vi "Output_file_Panel.vi"(8 "Show panel ?":bool, 9 "Channel Names":string[](array[string]), 10 "Header":string, 11 "Output filename":path=path "/G3_3 HD/Users/Paul/New Disp DB file") -> (0 "Save Full Res Data?":bool, 1 "Desired Columns":i32[](array[numeric]), 2 "Header Out":string, 3 "Output filename Out":path=path "/G3_3 HD/Users/Paul/New Disp DB file", 4 "Channels to Tabulate in header Out":i32[](listbox), 5 "Save Plotted rows only?":bool, 6 "Summarise mode":T1(ring), 7 "Grouping info":T3[](array[typedef]))   [LabVIEW 2010]
uses:
  Controls/Group_Binning.ctl
  Results_plotter_Global.vi
panel:
  in  "Channels to Tabulate in header":i32[](listbox)
  in  "Channels to first \"bin\" then output":i32[](listbox)
  in  "Channels to Ouput":i32[](listbox)
  out "Specified by Template":bool[](array[boolean])
  in  "Channel to bin":T2(array[cluster])
  in  "Summarize data":i32(listbox)=2
  in  "OK Button":bool
  in  "Column Selector":i32(listbox)
  in  "Row Selector":i32(listbox)=1
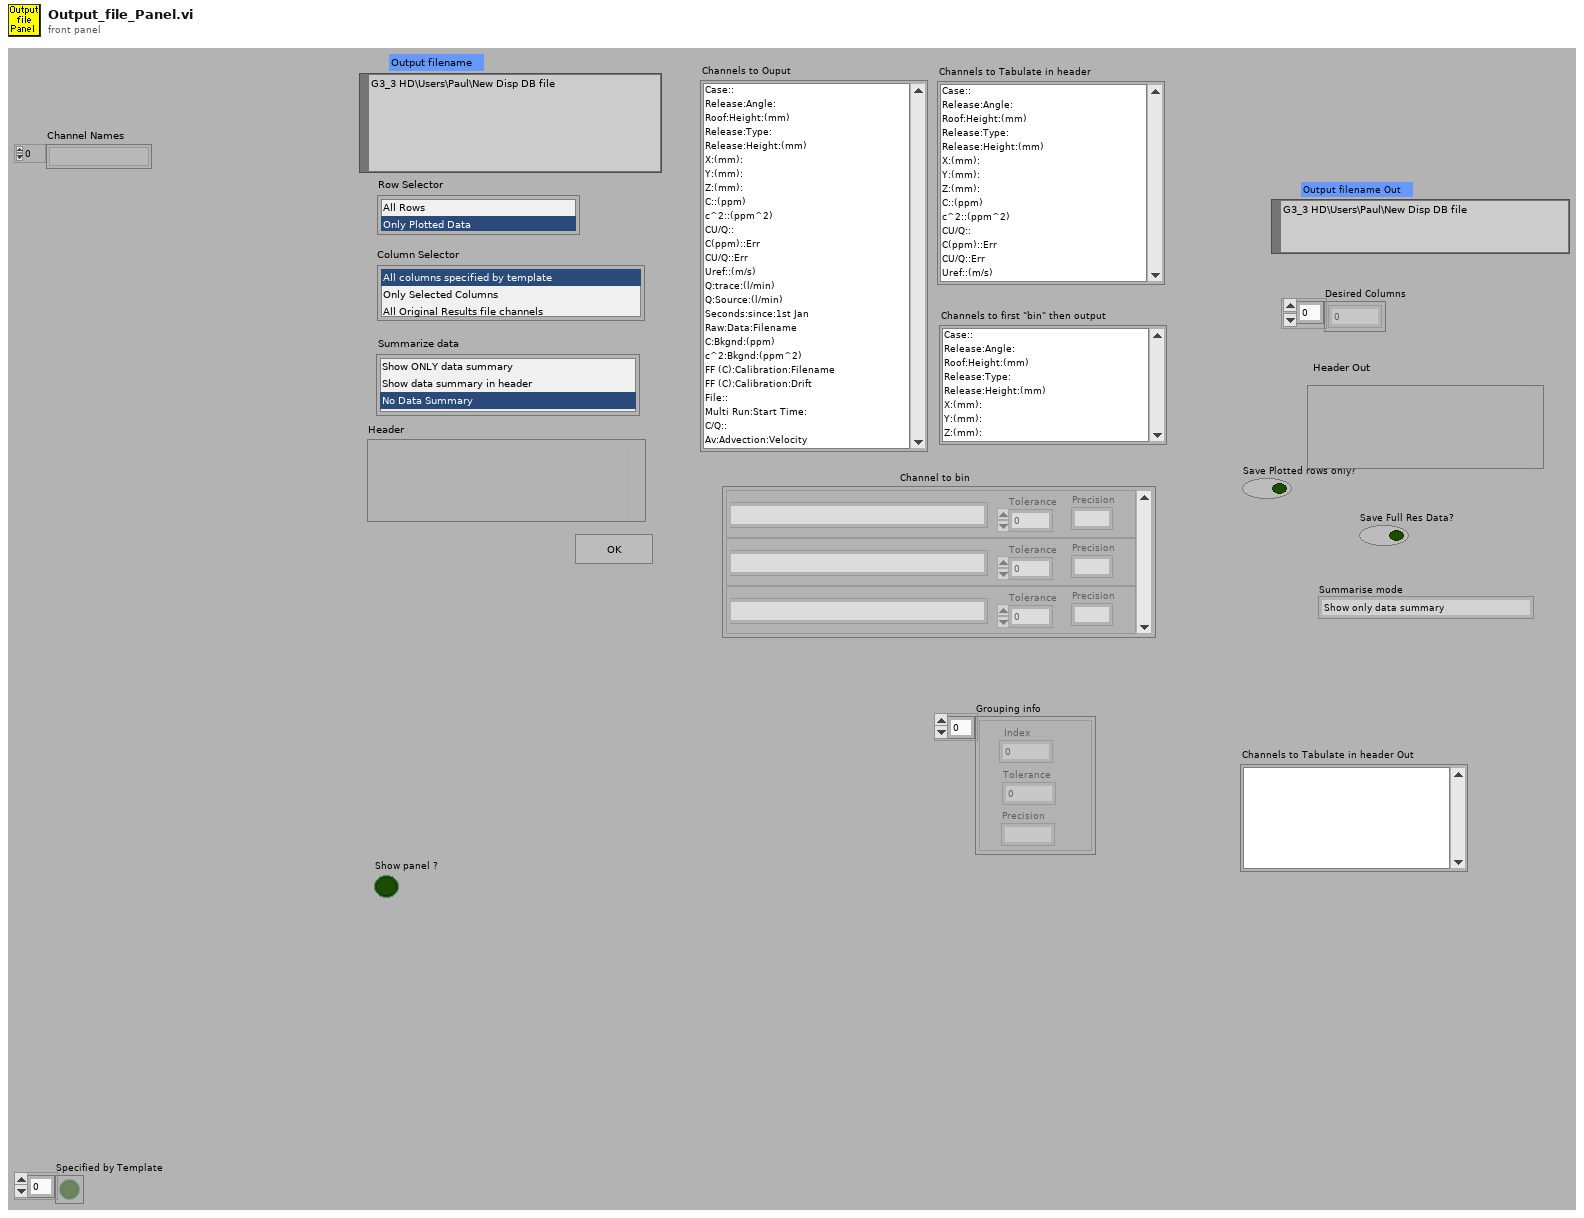
[diagram p1: front panel]
types:
  T1 = enum16{"Show only data summary", "Show data summary", "No data summary"}
  T2 = cluster{"Ch Name":string, "Tolerance":dbl, "Precision":string}[]
  T3 = typedef "Group_Binning.ctl" = cluster{"Index":i32, "Tolerance":dbl, "Precision":string}
  T4 = cluster{"Ch Name":string, "Tolerance":dbl, "Precision":string}
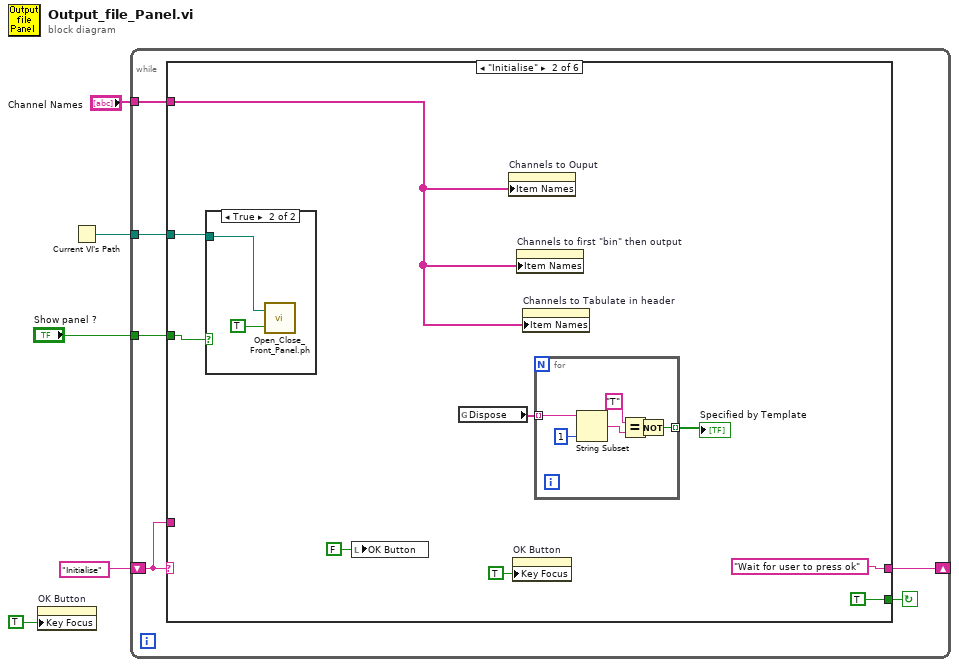
[diagram p0: block diagram]
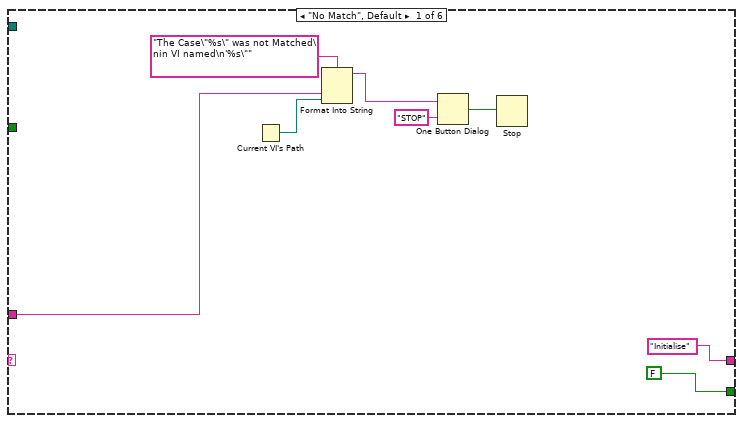
[diagram p2: hidden frame]
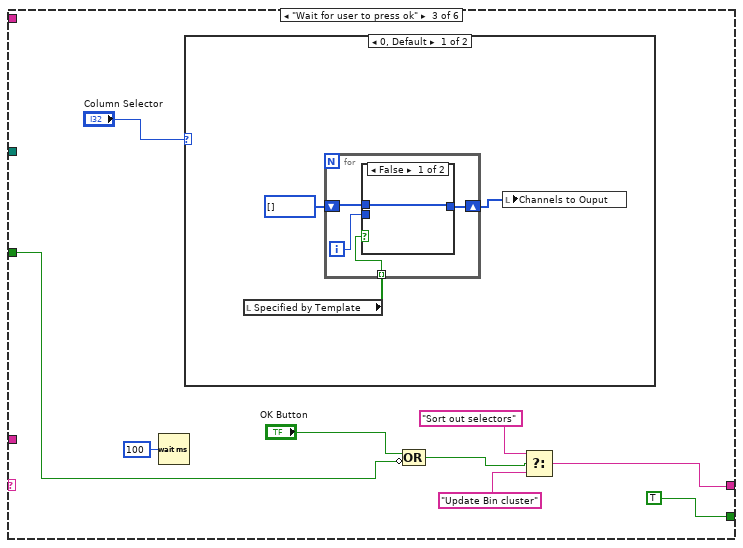
[diagram p4: hidden frame]
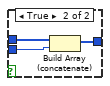
[diagram p5: hidden frame]
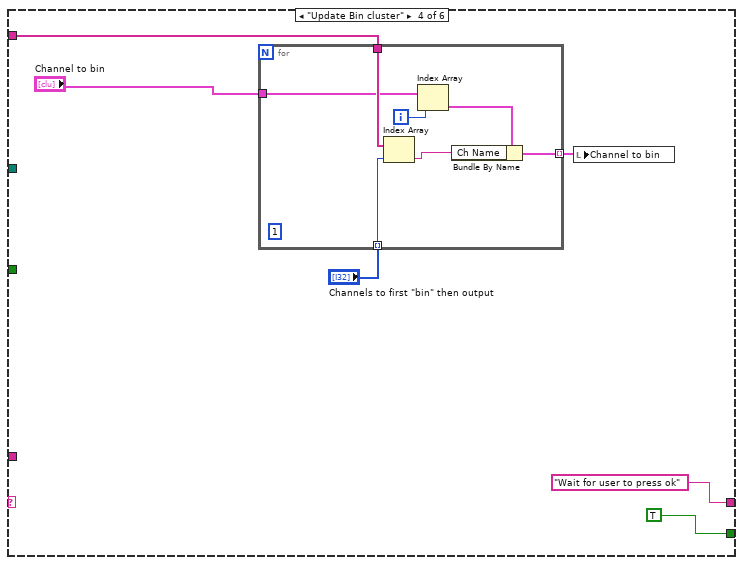
[diagram p7: hidden frame]
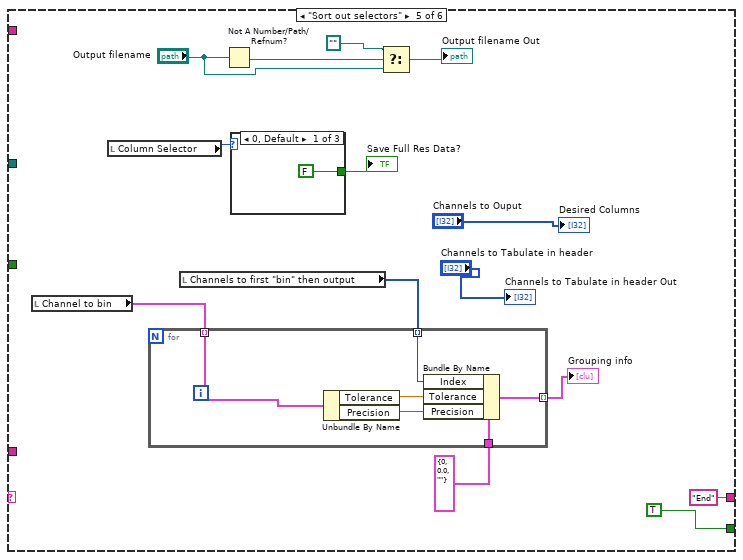
[diagram p8: hidden frame]
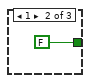
[diagram p9: hidden frame]
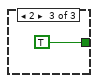
[diagram p10: hidden frame]
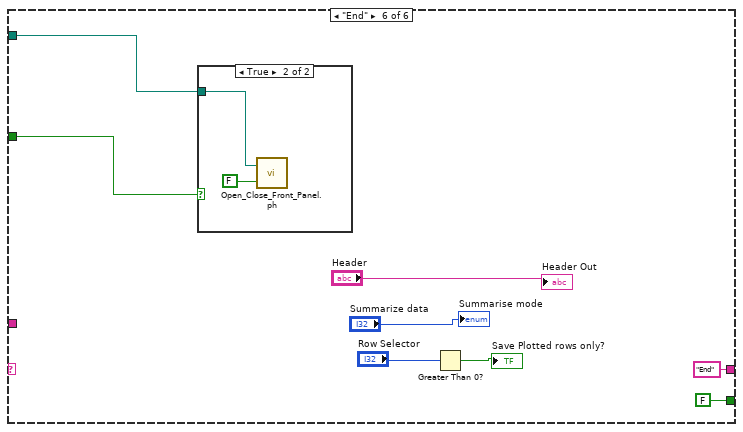
[diagram p11: hidden frame]
diagram:
  n1 = property on="OK Button" class="Bool (strict)"("Key Focus"=TRUE) -> ()  [unwired: 2 in, 2 out]
  n2 = Current VI's Path() -> (path=w3:path)
  n3 = while {
    shift-left: "Initialise" -> [w9]
    shift-right: [w10] -> _
    tunnel: "Show panel ?" -> [w8]
    tunnel: w3 -> [w7]
    tunnel: "Channel Names" -> [w6]
    stop <- w11 continue-if-true
    n4 = case shown="\"Initialise\"" w9 {
      tunnel: [FALSE TRUE TRUE TRUE TRUE FALSE] -> w11
      tunnel: ["Initialise" "Wait for user to press ok" w43 "Wait for user to press ok" "End" ("t") "End"] -> w10
      tunnel: w9 -> [w14 _ _ _ _ _]
      tunnel: w8 -> [_ w22 w37 _ _ w98]
      tunnel: w7 -> [_ w23 _ _ _ w97]
      tunnel: w6 -> [_ w24 _ w59 _ _]
      frame "No Match", Default {
        n5 = Current VI's Path() -> (path=w13:path)
        n6 = Format Into String(format string="The Case\"%s\" was not Matched\nin VI named\n'%s\"" ("Format String"), w14, w13) -> (resulting string=w17:string)  [unwired: 2 in, 1 out]
        n7 = One Button Dialog(message=w17, button name ("OK")="STOP") -> (true=w15:bool)
        n8 = Stop(stop? (T)=w15) -> ()
      }
      frame "Initialise" {
        n9 = case shown="True" w22 {
          tunnel: w23 -> [_ w30]
          frame False {
          }
          frame True {
            n10 = call "Open_Close_Front_Panel.ph.vi"("Front Panel Window:Open"=TRUE, "VI path"=w30) -> ()  [unwired: 2 out]
          }
        }
        n11 = local write "OK Button"(FALSE ("OK Button")) -> ()
        n12 = global read "Results_plotter_Global.vi" "Dispose"() -> (w28:string[])
        n13 = property on="Channels to Ouput" class="LstBox (strict)"("Item Names"=w24) -> ()  [unwired: 2 in, 2 out]
        n14 = property on="OK Button" class="Bool (strict)"("Key Focus"=TRUE) -> ()  [unwired: 2 in, 2 out]
        n15 = property on="Channels to first \"bin\" then output" class="LstBox (strict)"("Item Names"=w24) -> ()  [unwired: 2 in, 2 out]
        n16 = property on="Channels to Tabulate in header" class="LstBox (strict)"("Item Names"=w24) -> ()  [unwired: 2 in, 2 out]
        n17 = for {
          tunnel: w28 -> [w33] mode=indexing
          tunnel: [w31] -> w27 mode=indexing
          n18 = String Subset(string=w33, length (rest)=1 ("length (rest)")) -> (substring=w35:string)  [unwired: 1 out]
          n19 = Equal?(x="T", y=w35) -> (x = y?=w32:bool)
          n20 = Not(x=w32) -> (.not. x?=w31:bool)
        }
        "Specified by Template" <- w27
      }
      frame "Wait for user to press ok" {
        n21 = Wait (ms)(milliseconds to wait=u32 100) -> ()  [unwired: 1 out]
        n22 = case shown="0, Default" "Column Selector" {
          frame 0, Default {
            n23 = local read "Specified by Template"() -> (w48:bool[])
            n24 = for {
              shift-right: [w50] -> w46
              shift-left: i32[] [] -> [w51]
              tunnel: w48 -> [w52] mode=indexing
              i -> [w49]
              n25 = case shown="False" w52 {
                tunnel: w51 -> [w53 w56]
                tunnel: [w53 w55] -> w50
                tunnel: w49 -> [_ w54]
                frame False {
                }
                frame True {
                  n26 = Build Array (concatenate)(w56, w54) -> (w55:i32[])
                }
              }
            }
            n27 = local write "Channels to Ouput"(w46) -> ()
          }
          frame 1 {
          }
        }
        n28 = Compound Arithmetic op=OR("OK Button", invert w37) -> (w38:bool)
        n29 = Select(t="Sort out selectors", s=w38, f="Update Bin cluster") -> (s? t:f=w43:string)
      }
      frame "Update Bin cluster" {
        n30 = for {
          tunnel: "Channels to first \"bin\" then output" -> [w69] mode=indexing
          tunnel: w59 -> [w68]
          tunnel: "Channel to bin" -> [w65]
          tunnel: [w63] -> w57 mode=indexing
          i -> [w66]
          (unwired) 1 ("length (rest)")
          n31 = Index Array(array=w68, index=w69) -> (element=w67:string)
          n32 = Index Array(array=w65, index=w66) -> (element=w64:T4)
          n33 = Bundle By Name(cluster=w64, "Ch Name"=w67) -> (w63:T4)
        }
        n34 = local write "Channel to bin"(w57) -> ()
      }
      frame "Sort out selectors" {
        n35 = local read "Channel to bin"() -> (w75:T2)
        n36 = local read "Column Selector"() -> (w82:i32)
        n37 = local read "Channels to first \"bin\" then output"() -> (w72:i32[])
        n38 = for {
          tunnel: w75 -> [w89] mode=indexing
          tunnel: [w86] -> w74 mode=indexing
          tunnel: w72 -> [w85] mode=indexing
          tunnel: T3 {"Index"=0, "Tolerance"=0.0, "Precision"=""} ("Grouping info") -> [w84]
          n39 = Unbundle By Name(w89) -> ("Tolerance"=w88:dbl, "Precision"=w87:string)
          n40 = Bundle By Name(cluster=w84, "Index"=w85, "Tolerance"=w88, "Precision"=w87) -> (w86:T3)
        }
        "Grouping info" <- w74
        n41 = Not A Number/Path/Refnum?(number/path/refnum="Output filename") -> (NaN/Path/Refnum?=w79:bool)
        n42 = case shown="0, Default" w82 {
          tunnel: [FALSE FALSE TRUE] -> w80
          frame 0, Default {
          }
          frame 1 {
          }
          frame 2 {
          }
        }
        "Save Full Res Data?" <- w80
        n43 = Select(t=path "", s=w79, f="Output filename") -> (s? t:f=→"Output filename Out":path)
        "Desired Columns" <- "Channels to Ouput"
        "Channels to Tabulate in header Out" <- "Channels to Tabulate in header"
      }
      frame "End" {
        n44 = case shown="True" w98 {
          tunnel: w97 -> [_ w102]
          frame False {
          }
          frame True {
            n45 = call "Open_Close_Front_Panel.ph.vi"("Front Panel Window:Open"=FALSE, "VI path"=w102) -> ()  [unwired: 2 out]
          }
        }
        n46 = Greater Than 0?(x="Row Selector") -> (x > 0?=→"Save Plotted rows only?":bool)
        "Header Out" <- "Header"
        "Summarise mode" <- "Summarize data"
      }
    }
  }
